vi "DrawChessboardRadon.vi"(7 "Add Marker (Default: False)":bool, 8 "error in (no error)":errorcluster, 10 "Chessboard Corners Info":T4, 11 "Target Size":T3) -> (0 "error out":errorcluster, 3 "image data":T2)   [LabVIEW 2020, in "feature_detection.lvlib"]
uses:
  feature_detection.lvlib
  Chessboard Corner Info.ctl
  common/Image Size (Integer).ctl
  <vilib>/picture/picture.llb/imagedata.ctl
  common/Image Point (Integer).ctl
  ChessboardSquareLocation.ctl
  Chessboard Semi Circle Square Type.ctl
  Chessboard Teardrop Corner Type.ctl
  e7f4303d-582b-4721-b29a-aa63d9231187.vi
  <vilib>/picture/picture.llb/Draw Oval.vi
  <vilib>/Comparison/Equal/Equal Functor/Equal Functor.lvclass
  common/common.lvlib
panel:
  out "Origin Marker Square":T1
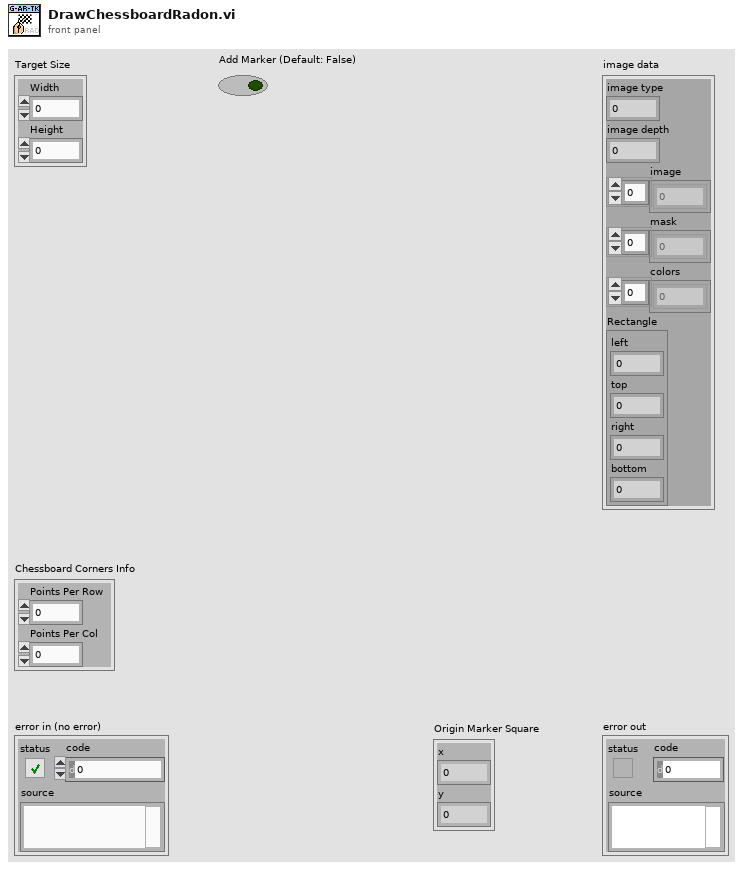
[diagram p1: front panel]
types:
  T1 = typedef "common.lvlib/Image Point (Integer).ctl" = cluster{"x":i32, "y":i32}
  T2 = typedef "imagedata.ctl" = cluster{"image type":i32, "image depth":i32, "image":u8[], "mask":u8[], "colors":u32[], "Rectangle":cluster{"left":i16, "top":i16, "right":i16, "bottom":i16}}
  T3 = typedef "common.lvlib/Image Size (Integer).ctl" = cluster{"Width":u16, "Height":u16}
  T4 = typedef "feature_detection.lvlib/Chessboard Corner Info.ctl" = cluster{"Points Per Row":u8, "Points Per Col":u8}
  T5 = cluster{"left":i16, "top":i16, "right":i16, "bottom":i16}
  T6 = typedef "feature_detection.lvlib/ChessboardSquareLocation.ctl" = enum16{"Top Left Corner", "Top Row", "Top Right Corner ", "Left Col", "Right Col", "Bottom Left Corner", "Bottom Row", "Bottom Right Corner", "Other"}
  T7 = map{cluster{"First Row":bool, "Last Row":bool, "First Col":bool, "Last Col":bool}, T6}
  T8 = cluster{"Points Per Row":i32, "Points Per Col":i32}
  T9 = cluster{"Points Per Row":i32, "Points Per Col":i32}[]
  T10 = cluster{"First Row":bool, "Last Row":bool, "First Col":bool, "Last Col":bool}
  T11 = cluster{"left":i32, "top":i32, "right":i32, "bottom":i32}
  T12 = typedef "feature_detection.lvlib/Chessboard Semi Circle Square Type.ctl" = enum16{"Top", "Left", "Right", "Bottom"}
  T13 = typedef "feature_detection.lvlib/Chessboard Teardrop Corner Type.ctl" = enum16{"Top Left", "Top Right", "Bottom Left", "Bottom Right"}
  T14 = cluster{"Width":i16, "Style":enum32{"Solid", "Dash", "Dot", "DashDot", "DashDotDot"}}
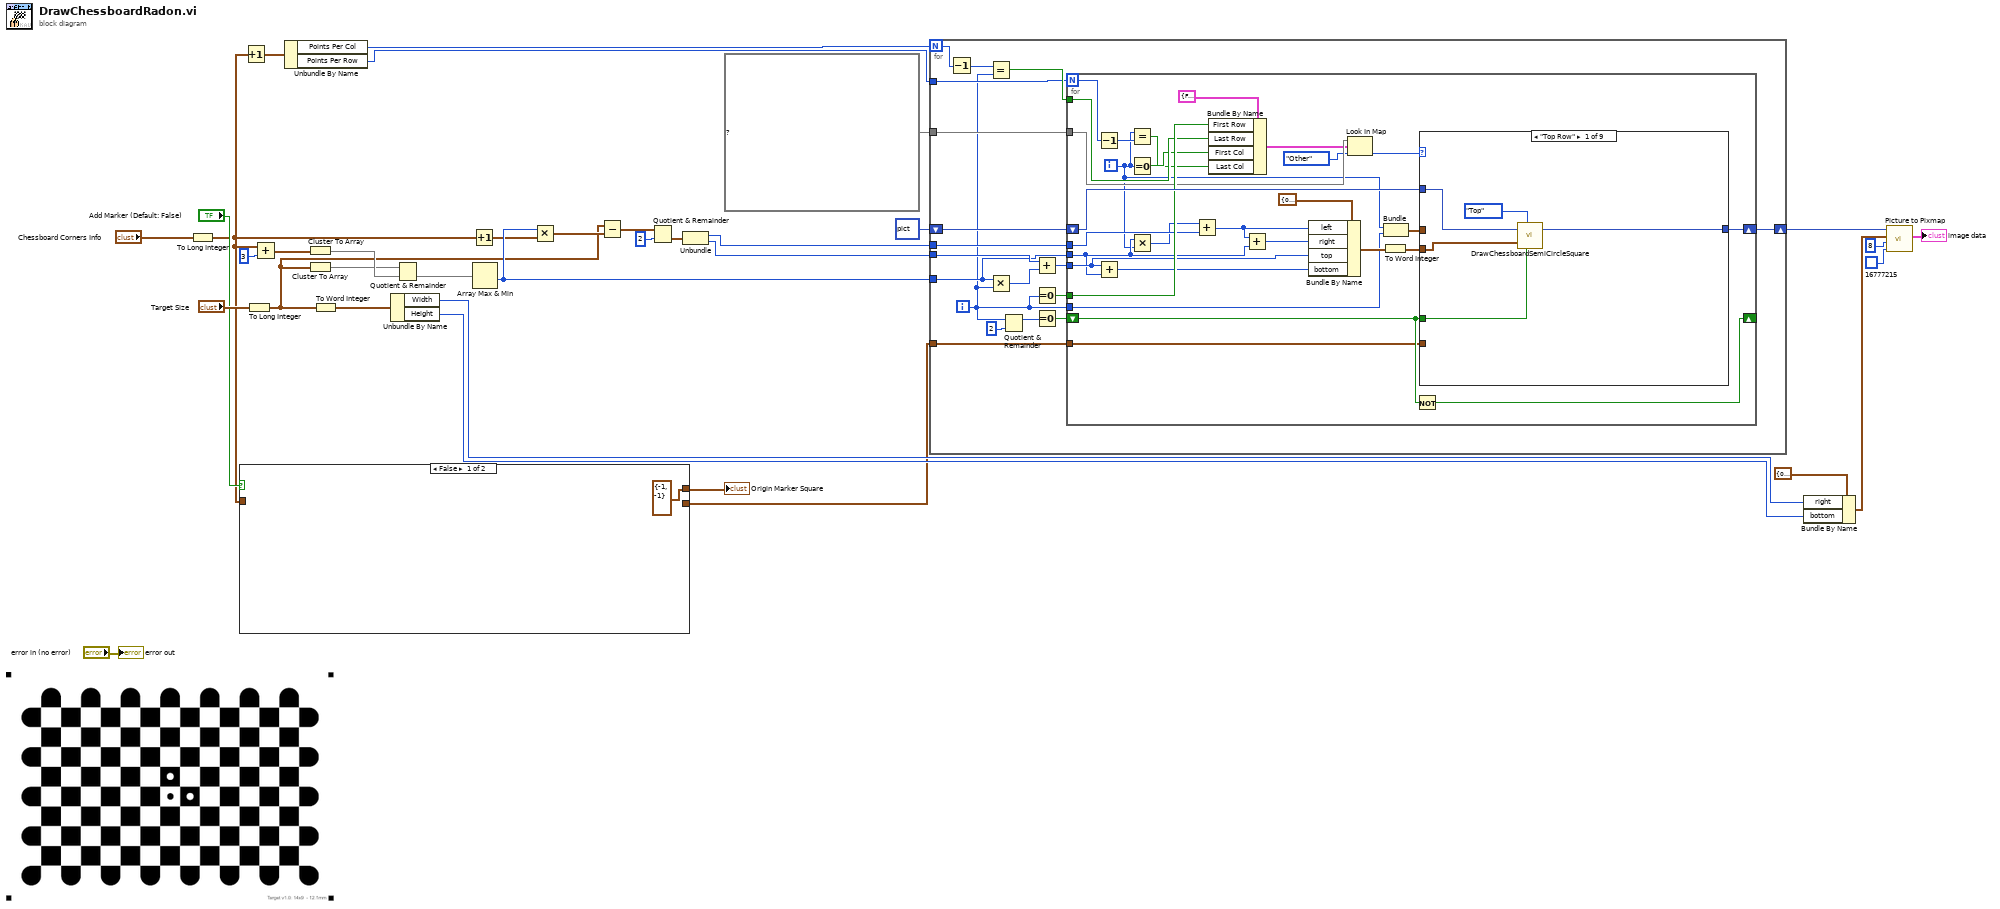
[diagram p0: block diagram]
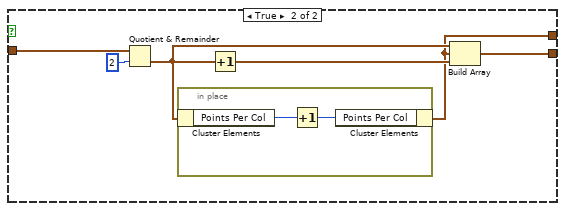
[diagram p2: hidden frame]
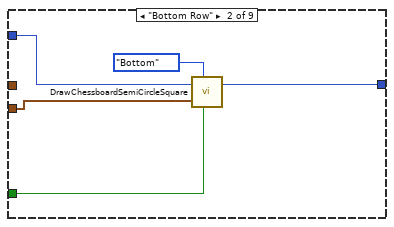
[diagram p3: hidden frame]
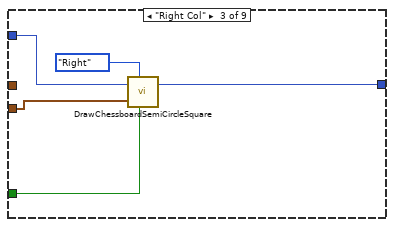
[diagram p4: hidden frame]
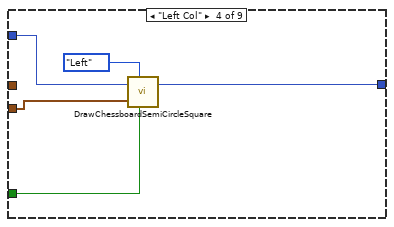
[diagram p5: hidden frame]
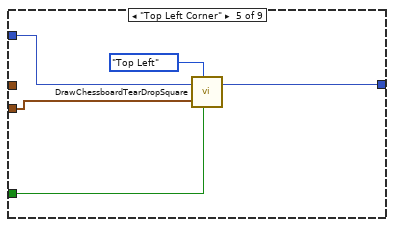
[diagram p6: hidden frame]
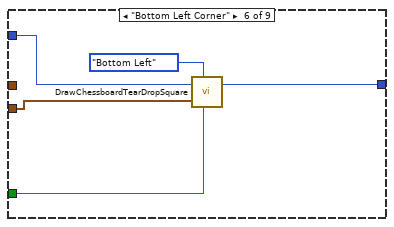
[diagram p7: hidden frame]
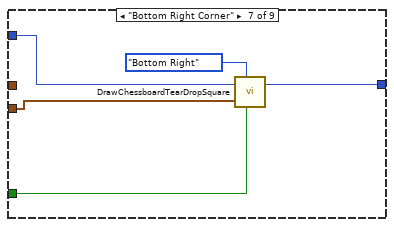
[diagram p8: hidden frame]
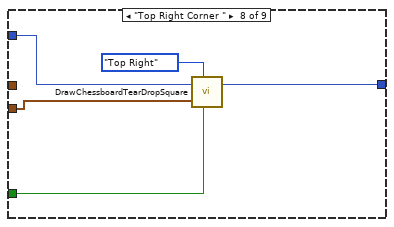
[diagram p9: hidden frame]
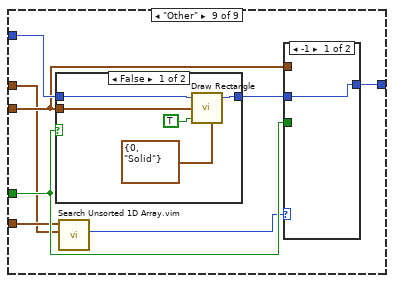
[diagram p10: hidden frame]
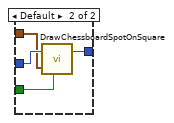
[diagram p11: hidden frame]
diagram:
  n1 = To Long Integer(number="Chessboard Corners Info") -> (32bit integer=w2:T8)
  n2 = case shown="False" "Add Marker (Default: False)" {
    tunnel: w2 -> [_ w42]
    tunnel: [_ w40] -> w3
    tunnel: [T8 {"Points Per Row"=-1, "Points Per Col"=-1} w37] -> w1
    frame False {
    }
    frame True {
      n3 = Quotient & Remainder(x=w42, y=2) -> (floor(x/y)=w39:T8)  [unwired: 1 out]
      n4 = in-place {
        n5 = in-place-cluster #1(w39) -> ("Points Per Col"=w44:i32)
        n6 = Increment(x=w44) -> (x+1=w43:i32)
        n7 = in-place-cluster #1("Points Per Col"=w43) -> (w37:T8)
      }
      n8 = Increment(x=w39) -> (x+1=w38:T8)
      n9 = Build Array(w39, w37, w38) -> (w40:T9)
    }
  }
  "Origin Marker Square" <- w1
  n10 = Increment(x=w2) -> (x+1=w5:T8)
  n11 = To Long Integer(number="Target Size") -> (32bit integer=w13:cluster{"Width":i32, "Height":i32})
  n12 = Add(x=w2, y=3) -> (x+y=w23:T8)
  n13 = Unbundle By Name(w5) -> ("Points Per Col"=w31:i32, "Points Per Row"=w6:i32)
  n14 = Cluster To Array(cluster=w23) -> (array=w15:i32[])
  n15 = Cluster To Array(cluster=w13) -> (array=w14:i32[])
  n16 = To Word Integer(number=w13) -> (16bit integer=w22:cluster{"Width":i16, "Height":i16})
  n17 = Unbundle By Name(w22) -> ("Width"=w28:i16, "Height"=w27:i16)
  n18 = Quotient & Remainder(x=w14, y=w15) -> (floor(x/y)=w33:i32[])  [unwired: 1 out]
  n19 = Increment(x=w2) -> (x+1=w17:T8)
  n20 = Array Max & Min(array=w33) -> (min value=w24:i32)  [unwired: 3 out]
  n21 = Multiply(x=w24, y=w17) -> (x*y=w21:T8)
  n22 = Subtract(x=w13, y=w21) -> (x-y=w20:cluster{i32, i32})
  n23 = Quotient & Remainder(x=w20, y=2) -> (floor(x/y)=w12:cluster{i32, i32})  [unwired: 1 out]
  n24 = Unbundle(w12) -> (w19:i32, w18:i32)
  n25 = for {
    N: w31 -> [w57]
    shift-right: [w61] -> w30
    shift-left: picture data[5B] ("picture") -> [w62]
    tunnel: w24 -> [w50]
    tunnel: w19 -> [w54]
    tunnel: w18 -> [w53]
    tunnel: T7 {{"First Row"=FALSE, "Last Row"=FALSE, "First Col"=FALSE, "Last Col"=TRUE}=enum."Right Col", {"First Row"=FALSE, "Last Row"=FALSE, "First Col"=TRUE, "Last Col"=FALSE}=enum."Left Col", {"First Row"=FALSE, "Last Row"=TRUE, "First Col"=FALSE, "Last Col"=FALSE}=enum."Bottom Row", {"First Row"=FALSE, "Last Row"=TRUE, "First Col"=FALSE, "Last Col"=TRUE}=enum."Bottom Right Corner", {"First Row"=FALSE, "Last Row"=TRUE, "First Col"=TRUE, "Last Col"=FALSE}=enum."Bottom Left Corner", {"First Row"=TRUE, "Last Row"=FALSE, "First Col"=FALSE, "Last Col"=FALSE}=enum."Top Row", {"First Row"=TRUE, "Last Row"=FALSE, "First Col"=FALSE, "Last Col"=TRUE}=enum."Top Right Corner ", {"First Row"=TRUE, "Last Row"=FALSE, "First Col"=TRUE, "Last Col"=FALSE}=enum."Top Left Corner"} ("Map") -> [w58]
    tunnel: w6 -> [w55]
    tunnel: w3 -> [w46]
    i -> [w45]
    n26 = Decrement(x=w57) -> (x-1=w56:i32)
    n27 = Equal?(x=w56, y=w45) -> (x = y?=w59:bool)
    n28 = Multiply(x=w50, y=w45) -> (x*y=w51:i32)
    n29 = Quotient & Remainder(x=w45, y=2) -> (x-y*floor(x/y)=w48:i32)  [unwired: 1 out]
    n30 = Add(x=w53, y=w51) -> (x+y=w52:i32)
    n31 = Equal To 0?(x=w45) -> (x = 0?=w60:bool)
    n32 = Equal To 0?(x=w48) -> (x = 0?=w47:bool)
    n33 = for {
      N: w55 -> [w80]
      shift-right: [w89] -> w61
      shift-left: w62 -> [w91]
      tunnel: w60 -> [w85]
      tunnel: w59 -> [w84]
      tunnel: w58 -> [w83]
      tunnel: w50 -> [w70]
      tunnel: w54 -> [w73]
      tunnel: w52 -> [w72]
      shift-right: [w68] -> _
      shift-left: w47 -> [w67]
      tunnel: w46 -> [w66]
      tunnel: w45 -> [w63]
      i -> [w64]
      n34 = Decrement(x=w80) -> (x-1=w79:i32)
      n35 = Add(x=w72, y=w70) -> (x+y=w77:i32)
      n36 = Equal?(x=w64, y=w79) -> (x = y?=w74:bool)
      n37 = Equal To 0?(x=w64) -> (x = 0?=w75:bool)
      n38 = Multiply(x=w70, y=w64) -> (x*y=w69:i32)
      n39 = Add(x=w69, y=w73) -> (x+y=w71:i32)
      n40 = Bundle By Name(cluster=T10 {"First Row"=FALSE, "Last Row"=FALSE, "First Col"=FALSE, "Last Col"=FALSE} ("Position"), "First Row"=w85, "Last Row"=w84, "First Col"=w75, "Last Col"=w74) -> (w82:T10)
      n41 = Add(x=w71, y=w70) -> (x+y=w78:i32)
      n42 = Bundle By Name(cluster=T11 {"left"=0, "top"=0, "right"=0, "bottom"=0} ("32bit integer"), "left"=w71, "right"=w78, "top"=w72, "bottom"=w77) -> (w90:T11)
      n43 = Look In Map(map=w83, key=w82, default value=ChessboardSquareLocation."Other") -> (value=w76:T6)  [unwired: 1 out]
      n44 = To Word Integer(number=w90) -> (16bit integer=w88:T5)
      n45 = Bundle(w64, w63) -> (w65:cluster{i32, i32})  [unwired: 1 in]
      n46 = Not(x=w67) -> (.not. x?=w68:bool)
      n47 = case shown="\"Top Row\"" w76 {
        tunnel: w91 -> [w96 w101 w106 w111 w116 w121 w126 w131 w139]
        tunnel: [w95 w100 w105 w110 w115 w120 w125 w130 w137] -> w89
        tunnel: w88 -> [w94 w99 w104 w109 w114 w119 w124 w129 w135]
        tunnel: w67 -> [w92 w97 w102 w107 w112 w117 w122 w127 w136]
        tunnel: w66 -> [_ _ _ _ _ _ _ _ w134]
        tunnel: w65 -> [_ _ _ _ _ _ _ _ w133]
        frame "Top Row" {
          n48 = call "DrawChessboardSemiCircleSquare.vi"("Bounds"=w94, "Skip"=w92, "picture in"=w96, "Semi Circle Square Type"=Chessboard_Semi_Circle_Square_Type."Top") -> ("picture out"=w95:picture)  [unwired: 3 in]
        }
        frame "Bottom Row" {
          n49 = call "DrawChessboardSemiCircleSquare.vi"("Bounds"=w99, "Skip"=w97, "picture in"=w101, "Semi Circle Square Type"=Chessboard_Semi_Circle_Square_Type."Bottom") -> ("picture out"=w100:picture)  [unwired: 3 in]
        }
        frame "Right Col" {
          n50 = call "DrawChessboardSemiCircleSquare.vi"("Bounds"=w104, "Skip"=w102, "picture in"=w106, "Semi Circle Square Type"=Chessboard_Semi_Circle_Square_Type."Right") -> ("picture out"=w105:picture)  [unwired: 3 in]
        }
        frame "Left Col" {
          n51 = call "DrawChessboardSemiCircleSquare.vi"("Bounds"=w109, "Skip"=w107, "picture in"=w111, "Semi Circle Square Type"=Chessboard_Semi_Circle_Square_Type."Left") -> ("picture out"=w110:picture)  [unwired: 3 in]
        }
        frame "Top Left Corner" {
          n52 = call "DrawChessboardTearDropSquare.vi"("Bounds"=w114, "Skip"=w112, "picture in"=w116, "Tear Drop Corner"=Chessboard_Teardrop_Corner_Type."Top Left") -> ("picture out"=w115:picture)  [unwired: 3 in]
        }
        frame "Bottom Left Corner" {
          n53 = call "DrawChessboardTearDropSquare.vi"("Bounds"=w119, "Skip"=w117, "picture in"=w121, "Tear Drop Corner"=Chessboard_Teardrop_Corner_Type."Bottom Left") -> ("picture out"=w120:picture)  [unwired: 3 in]
        }
        frame "Bottom Right Corner" {
          n54 = call "DrawChessboardTearDropSquare.vi"("Bounds"=w124, "Skip"=w122, "picture in"=w126, "Tear Drop Corner"=Chessboard_Teardrop_Corner_Type."Bottom Right") -> ("picture out"=w125:picture)  [unwired: 3 in]
        }
        frame "Top Right Corner " {
          n55 = call "DrawChessboardTearDropSquare.vi"("Bounds"=w129, "Skip"=w127, "picture in"=w131, "Tear Drop Corner"=Chessboard_Teardrop_Corner_Type."Top Right") -> ("picture out"=w130:picture)  [unwired: 3 in]
        }
        frame "Other" {
          n56 = case shown="False" w136 {
            tunnel: w139 -> [w149 w150]
            tunnel: [w148 w150] -> w138
            tunnel: w135 -> [w147 _]
            frame False {
              n57 = call <vilib>:"Draw Rectangle.vi"("picture"=w149, "rect"=w147, "fill?(F)"=TRUE, "pen"=T14 {"Width"=0, "Style"=enum."Solid"}) -> ("new picture"=w148:picture)  [unwired: 5 in]
            }
            frame True {
            }
          }
          n58 = call "Search Unsorted 1D Array.vim"("element"=w133, "unsorted 1D array"=w134) -> ("index of element"=w132:i32)  [unwired: 9 in]
          n59 = case shown="-1" w132 {
            tunnel: w138 -> [w140 w144]
            tunnel: [w140 w143] -> w137
            tunnel: w136 -> [_ w142]
            tunnel: w135 -> [_ w141]
            frame -1 {
            }
            frame Default {
              n60 = call "DrawChessboardSpotOnSquare.vi"("Bounds"=w141, "Black On White"=w142, "picture in"=w144) -> ("picture out"=w143:picture)  [unwired: 4 in]
            }
          }
        }
      }
    }
  }
  n61 = Bundle By Name(cluster=T5 {"left"=0, "top"=0, "right"=0, "bottom"=0} ("rect"), "right"=w28, "bottom"=w27) -> (w16:T5)
  n62 = call <vilib>:"Picture to Pixmap.vi"("Background Color"=u32 16777215, "depth"=8, "rect"=w16, "picture"=w30) -> ("image data"=→"image data":T2)  [unwired: 6 in, 1 out]
  "error out" <- "error in (no error)"
